vi "SCM4_PS_Control_Remote.vi"() -> ()   [LabVIEW 2018]
panel:
  in  "Slew rate":dbl=1.0 format="%#_4g"
  out "error out 3":errorcluster
  in  "Setpoint":dbl format="%#_4g"
  in  "stop":bool
  in  "port":u16=3377
  in  "error in (no error) 2":errorcluster
  in  "Data mac ip address":string="146.201.201.20"
  out "Field [T]":dbl=-17.9883723 format="%#_4g"
  # "[T/min]"
  # "Note\n(1) Exception of the firewall should be configured.\n(2) With some (not all) connection with PC's, it is successful only when the VI is first executed. If the VI is stopped (normally or by aborting), \nthe subsequent connection is only possible with a new port number."
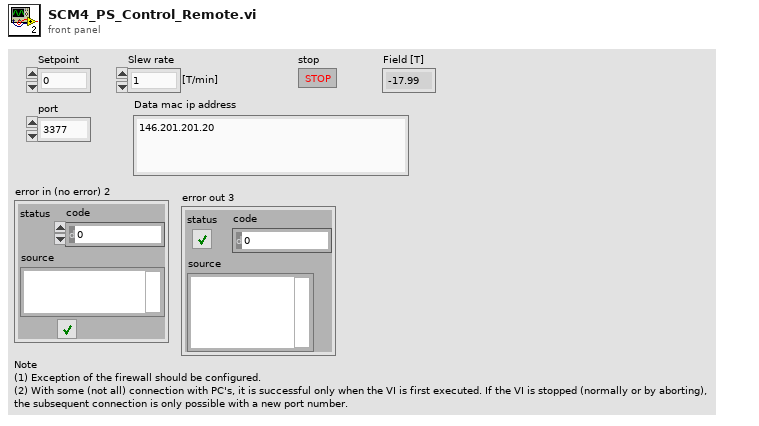
[diagram p1: front panel]
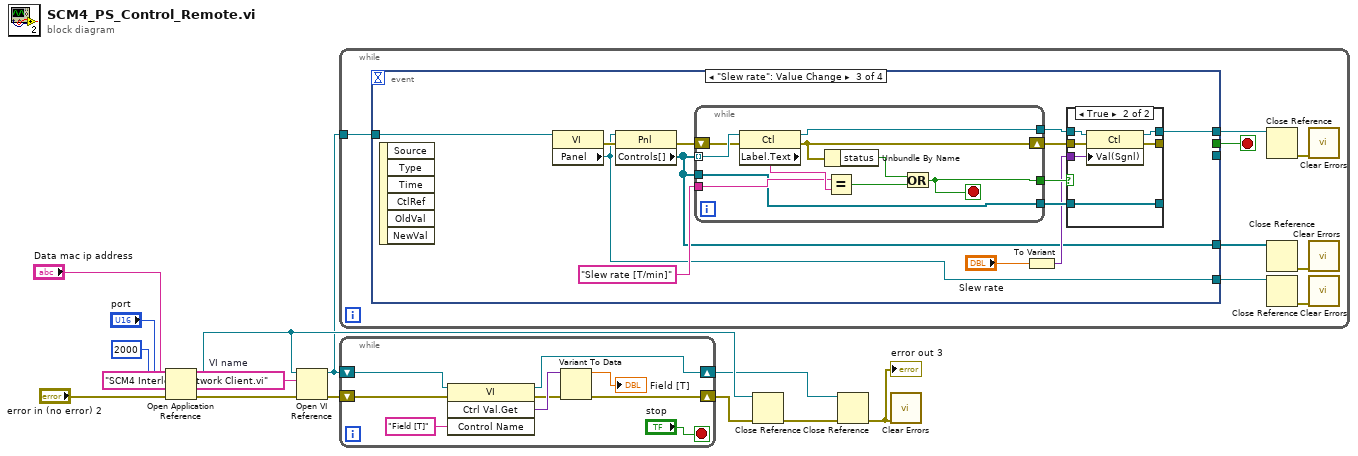
[diagram p0: block diagram]
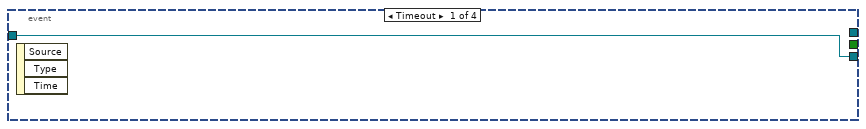
[diagram p2: hidden frame]
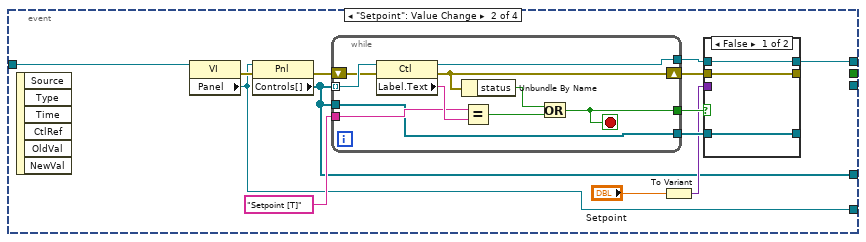
[diagram p3: hidden frame]
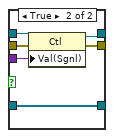
[diagram p4: hidden frame]
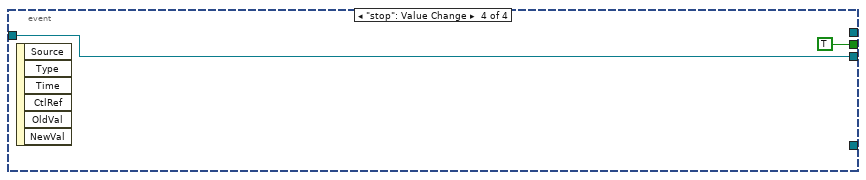
[diagram p6: hidden frame]
diagram:
  w5 = "SCM4 Interlock Network Client.vi"  # VI name
  n1 = Open Application Reference(8:"error in (no error) 2", 9:2000 ("timeout ms (60000)"), 10:"port", 11:"Data mac ip address") -> (0:w12:errorcluster, 3:w7:refnum<vi>)
  n2 = Open VI Reference(application reference (local)=w7, vi path=w5, error in (no error)=w12) -> (vi reference=w2:refnum<vi>, error out=w1:errorcluster)  [unwired: 3 in]
  n3 = while {
    tunnel: w2 -> [w17]
    stop <- w21 stop-if-true
    n4 = event shown="[2] \"Slew rate\": Value Change" {
      selector: _ -> [_ _ _ _]
      dyn-events: _ -> [_ _ _ _]
      timeout: _ -> [_ _ _ _]
      tunnel: w17 -> [w22 w26 w59 w87]
      tunnel: [_ _ _ TRUE] -> w21
      tunnel: [w22 _ _ w87] -> _
      tunnel: [_ w25 w58 _] -> w20
      tunnel: [_ w24 w57 _] -> w18
      tunnel: [_ w23 w55 _] -> w19
      event Timeout {
        n5 = event-data() -> ()  [unwired: 1 in, 3 out]
      }
      event "Setpoint": Value Change {
        n6 = event-data() -> ()  [unwired: 1 in, 6 out]
        n7 = property class="VI"(reference=w26) -> (error out=w35:errorcluster, "Panel"=w24:refnum<vi>)  [unwired: 1 in, 1 out]
        n8 = property class="Pnl"(reference=w24, error in=w35) -> (error out=w34:errorcluster, "Controls[]"=w25:refnum<vi>[])  [unwired: 1 out]
        n9 = while {
          tunnel: w25 -> [w54] mode=indexing
          tunnel: "Setpoint [T]" ("Control Name") -> [w52]
          shift-right: [w49] -> w31
          shift-left: w34 -> [w51]
          tunnel: [w50] -> w33
          tunnel: [w46] -> w32
          tunnel: w25 -> [w45]
          tunnel: [w45] -> w30
          stop <- w46 stop-if-true
          n10 = property class="Ctl"(reference=w54, error in=w51) -> (reference out=w50:refnum<vi>, error out=w49:errorcluster, "Label.Text"=w53:string)
          n11 = Unbundle By Name(w49) -> ("status"=w48:bool)
          n12 = Equal?(x=w52, y=w53) -> (x = y?=w47:bool)
          n13 = Or(x=w48, y=w47) -> (x .or. y?=w46:bool)
        }
        n14 = To Variant(anything="Setpoint") -> (Variant=w27:variant)
        n15 = case shown="False" w32 {
          tunnel: w33 -> [w37 w43]
          tunnel: w31 -> [w38 w44]
          tunnel: [w38 w42] -> _
          tunnel: [w37 w41] -> w23
          tunnel: w30 -> [w36 w40]
          tunnel: [w36 w40] -> _
          tunnel: w27 -> [_ w39]
          frame False {
          }
          frame True {
            n16 = property class="Ctl"(reference=w43, error in=w44, "Val(Sgnl)"=w39) -> (reference out=w41:refnum<vi>, error out=w42:errorcluster)
          }
        }
      }
      event "Slew rate": Value Change {
        n17 = event-data() -> ()  [unwired: 1 in, 6 out]
        n18 = property class="VI"(reference=w59) -> (error out=w67:errorcluster, "Panel"=w57:refnum<vi>)  [unwired: 1 in, 1 out]
        n19 = property class="Pnl"(reference=w57, error in=w67) -> (error out=w66:errorcluster, "Controls[]"=w58:refnum<vi>[])  [unwired: 1 out]
        n20 = while {
          tunnel: w58 -> [w86] mode=indexing
          tunnel: "Slew rate [T/min]" ("Control Name") -> [w84]
          shift-right: [w81] -> w63
          shift-left: w66 -> [w83]
          tunnel: [w82] -> w65
          tunnel: [w78] -> w64
          tunnel: w58 -> [w77]
          tunnel: [w77] -> w62
          stop <- w78 stop-if-true
          n21 = property class="Ctl"(reference=w86, error in=w83) -> (reference out=w82:refnum<vi>, error out=w81:errorcluster, "Label.Text"=w85:string)
          n22 = Unbundle By Name(w81) -> ("status"=w80:bool)
          n23 = Equal?(x=w84, y=w85) -> (x = y?=w79:bool)
          n24 = Or(x=w80, y=w79) -> (x .or. y?=w78:bool)
        }
        n25 = To Variant(anything="Slew rate") -> (Variant=w60:variant)
        n26 = case shown="True" w64 {
          tunnel: w65 -> [w69 w75]
          tunnel: w63 -> [w70 w76]
          tunnel: [w70 w74] -> _
          tunnel: [w69 w73] -> w55
          tunnel: w62 -> [w68 w72]
          tunnel: [w68 w72] -> _
          tunnel: w60 -> [_ w71]
          frame False {
          }
          frame True {
            n27 = property class="Ctl"(reference=w75, error in=w76, "Val(Sgnl)"=w71) -> (reference out=w73:refnum<vi>, error out=w74:errorcluster)
          }
        }
      }
      event "stop": Value Change {
        n28 = event-data() -> ()  [unwired: 1 in, 6 out]
      }
    }
    n29 = Close Reference(reference=w19) -> (error out=w14:errorcluster)  [unwired: 1 in]
    n30 = Close Reference(reference=w20) -> (error out=w15:errorcluster)  [unwired: 1 in]
    n31 = Close Reference(reference=w18) -> (error out=w16:errorcluster)  [unwired: 1 in]
    n32 = call <vilib>:"Clear Errors.vi"("error in (no error)"=w14) -> ()  [unwired: 5 in, 2 out]
    n33 = call <vilib>:"Clear Errors.vi"("error in (no error)"=w15) -> ()  [unwired: 5 in, 2 out]
    n34 = call <vilib>:"Clear Errors.vi"("error in (no error)"=w16) -> ()  [unwired: 5 in, 2 out]
  }
  n35 = while {
    shift-right: [w95] -> w6
    shift-left: w2 -> [w90]
    shift-right: [w97] -> w9
    shift-left: w1 -> [w89]
    stop <- "stop" stop-if-true
    n36 = invoke class="VI" method="Ctrl Val.Get"(reference=w90, error in=w89, "Control Name"="Field [T]") -> (reference out=w95:refnum<vi>, error out=w93:errorcluster, "Get Control Value Variant"=w94:variant)  [unwired: 1 in, 1 out]
    n37 = Variant To Data(error in=w93, Variant=w94) -> (data=→"Field [T]":dbl, error out=w97:errorcluster)  [unwired: 1 in]
  }
  n38 = Close Reference(reference=w7, error in (no error)=w9) -> (error out=w8:errorcluster)
  n39 = Close Reference(reference=w6, error in (no error)=w8) -> (error out=w3:errorcluster)
  "error out 3" <- w3
  n40 = call <vilib>:"Clear Errors.vi"("error in (no error)"=w3) -> ()  [unwired: 5 in, 2 out]
